vi "Get Byte Stream Info.vi"(8 "error in (no error)":errorcluster, 11 "Mapped-Buffer":refnum<class "Buffer Byte-Stream Access.lvclass">) -> (0 "error out":errorcluster, 1 "Byte Stream (Do Not Delete)":refnum<data-value>, 2 "Y Resolution":i32, 3 "X Resolution":i32, 4 "Bytes to Copy":u64)   [LabVIEW 2020, in "Buffer Byte-Stream Access.lvclass"]
uses:
  Buffer Byte-Stream Access.lvclass
  Buffer Byte-Stream Access.lvclass/Buffer Byte-Stream Access.ctl
  Buffer/Buffer.lvclass/Buffer.ctl
  Buffer/Buffer.lvclass
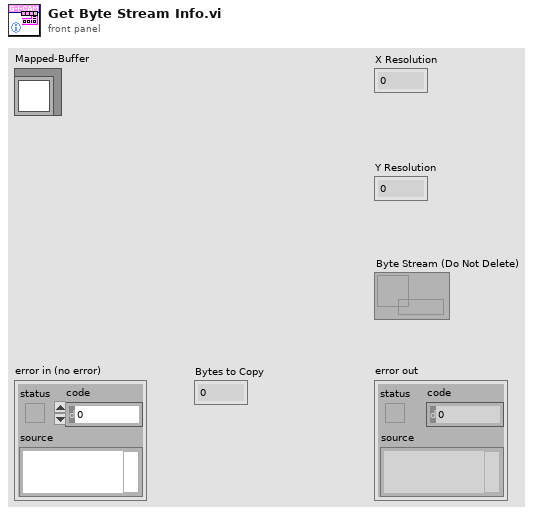
[diagram p1: front panel]
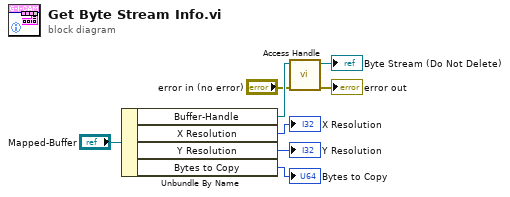
[diagram p0: block diagram]
diagram:
  n1 = Unbundle By Name("Mapped-Buffer") -> ("Buffer-Handle"=w4:refnum<class "Buffer.lvclass">, "X Resolution"=→"X Resolution":i32, "Y Resolution"=→"Y Resolution":i32, "Bytes to Copy"=→"Bytes to Copy":u64)
  n2 = call "Access Handle.vi"("error in (no error)"="error in (no error)", "Buffer"=w4) -> ("error out"=→"error out":errorcluster, "Handle"=→"Byte Stream (Do Not Delete)":refnum<data-value>)  [unwired: 8 in]
